vi "CC Script Send Script Start Status.vi"(8 "error in (no error)":errorcluster, 11 "Data Q":refnum<queue>) -> (0 "error out":errorcluster)   [LabVIEW 2024]
uses:
  Subsystems/SS cluster Data Queue type.ctl
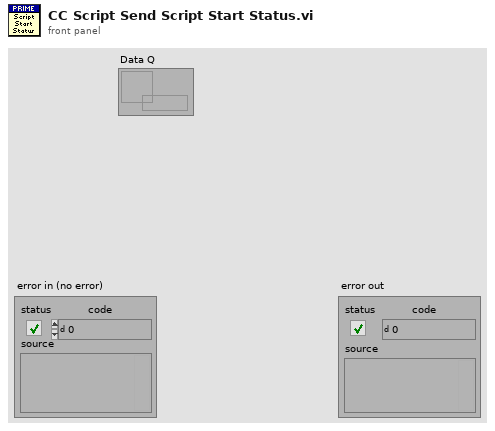
[diagram p1: front panel]
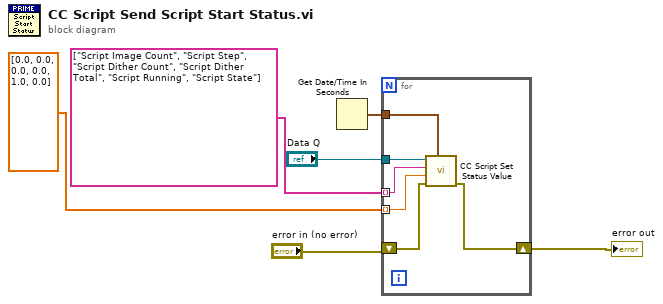
[diagram p0: block diagram]
diagram:
  n1 = Get Date/Time In Seconds() -> (seconds since 1Jan1904=w3:timestamp)
  n2 = for {
    tunnel: "Data Q" -> [w12]
    tunnel: string[] ["Script Image Count", "Script Step", "Script Dither Count", "Script Dither Total", "Script Running", "Script State"] -> [w11] mode=indexing
    tunnel: dbl[] [0.0, 0.0, 0.0, 0.0, 1.0, 0.0] -> [w10] mode=indexing
    tunnel: w3 -> [w9]
    shift-right: [w7] -> w1
    shift-left: "error in (no error)" -> [w8]
    n3 = call "CC Script Set Status Value.vi"("Time Stamp"=w9, "error in (no error)"=w8, "Value"=w10, "Ch Name"=w11, "Data Q"=w12) -> ("error out"=w7:errorcluster)  [unwired: 6 in]
  }
  "error out" <- w1
